vi "Get Flash Positions.vi"(11 "Grid In":i64[][](array[numeric])) -> (3 "Flash Positions":cluster{"X":i32, "Y":i32}[](array[cluster]))   [LabVIEW 2021]
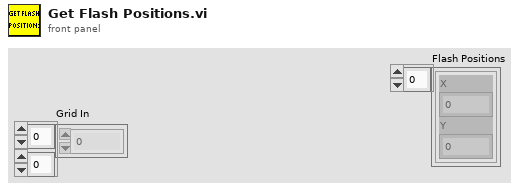
[diagram p1: front panel]
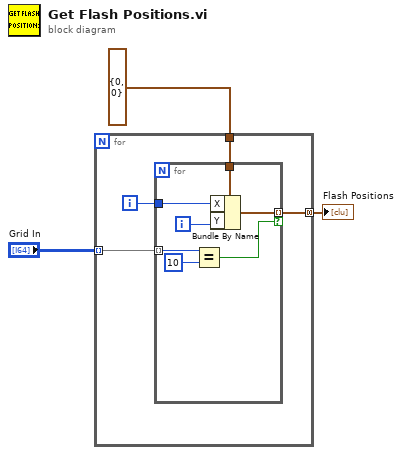
[diagram p0: block diagram]
diagram:
  n1 = for {
    tunnel: "Grid In" -> [w7] mode=indexing
    tunnel: cluster{"X":i32, "Y":i32} {"X"=0, "Y"=0} -> [w6]
    tunnel: [w4] -> w1 mode=concatenating
    i -> [w5]
    n2 = for {
      tunnel: w7 -> [w14] mode=indexing
      tunnel: w6 -> [w11]
      tunnel: w5 -> [w10]
      tunnel: [w9] -> w4 mode=indexing if=w8
      i -> [w12]
      n3 = Equal?(x=w14, y=i64 10) -> (x = y?=w8:bool)
      n4 = Bundle By Name(cluster=w11, "X"=w10, "Y"=w12) -> (w9:cluster{"X":i32, "Y":i32})
    }
  }
  "Flash Positions" <- w1
